vi "WriteExternalInterfaces.vi"(8 "ErrorIn":errorcluster, 10 "ExternalInterfaces":T1[](array[typedef]), 11 "OpenCVFaceDetectionIn":refnum<class "OpenCVFaceDetection.lvclass">) -> (0 "ErrorOut":errorcluster, 3 "OpenCVFaceDetectionOut":refnum<class "OpenCVFaceDetection.lvclass">)   [LabVIEW 2021, in "OpenCVFaceDetection.lvclass"]
uses:
  OpenCVFaceDetection.lvclass
  .Externals/Library_TAF_Support/ClusterArrayConversion/BundledArray.ctl
  OpenCVFaceDetection.lvclass/OpenCVFaceDetection.ctl
  0f9fbe56-9f9a-4601-8b43-1fc07a995cee.vi
  0f9fbe56-9f9a-4601-8b43-1fc07a995cee.vi/e733eca7-9823-4359-8665-3b184f9a7377.vi
  0f9fbe56-9f9a-4601-8b43-1fc07a995cee.vi/185eb5ab-e8f7-4395-854b-f566a9b9020c.vi
  <vilib>/Utility/Data Type/Get Cluster Information.vi
  <vilib>/Utility/Data Type/Get Type Information.vi
  <userlib>/_OpenG.lib/lvdata/lvdata.llb/Array of VData to VCluster__ogtk.vi
  <vilib>/Utility/LVClass/Get LV Class Name.vi
  .Externals/Library_TAF_Support/ClusterArrayConversion/ClusterArrayConversion.lvlib
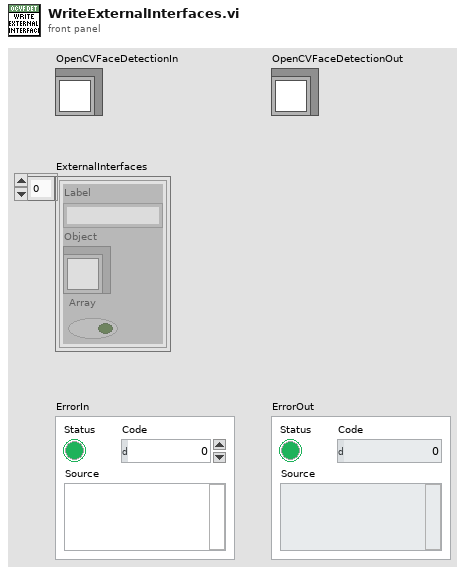
[diagram p1: front panel]
types:
  T1 = typedef "ClusterArrayConversion.lvlib/BundledArray.ctl" = cluster{"Label":string, "Object":refnum<class>, "Array":bool}
  T2 = cluster{"TAFObject":refnum<class "ITAFObject.lvclass">}
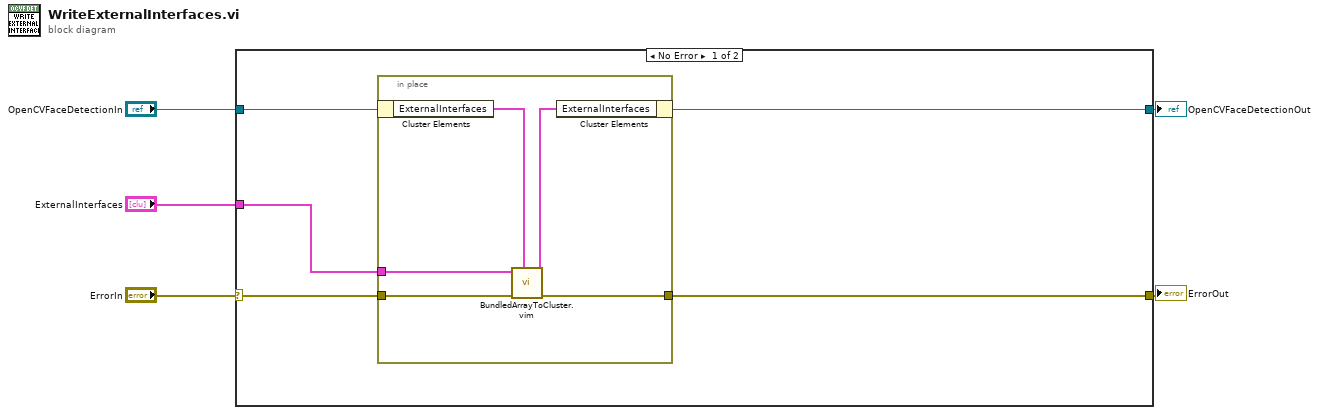
[diagram p0: block diagram]
diagram:
  n1 = case shown="No Error" "ErrorIn" {
    selector: "ErrorIn" -> [w10 w17]
    tunnel: [w9 w17] -> w4
    tunnel: [w6 w16] -> w2
    tunnel: "OpenCVFaceDetectionIn" -> [w8 w16]
    tunnel: "ExternalInterfaces" -> [w7 _]
    frame No Error {
      n2 = in-place {
        in-place-border: [w15] -> w9
        in-place-border: w10 -> [w14]
        in-place-border: w7 -> [w13]
        n3 = in-place-cluster #1(w8) -> ("ExternalInterfaces"=w12:T2)
        n4 = call "BundledArrayToCluster.vim"("Type"=w12, "ErrorIn"=w14, "BundeledLabels"=w13) -> ("ErrorOut"=w15:errorcluster, "DataOut"=w11:T2)  [unwired: 7 in]
        n5 = in-place-cluster #1("ExternalInterfaces"=w11) -> (w6:refnum<class "OpenCVFaceDetection.lvclass">)
      }
    }
    frame Error {
    }
  }
  "ErrorOut" <- w4
  "OpenCVFaceDetectionOut" <- w2
